vi "People Position to Steering Velocity.vi"(6 "image resolution":cluster{"x":i32, "y":i32}={"x"=640, "y"=480}, 8 "error in (no error)":errorcluster, 10 "ball pixel position":T1, 11 "ball found?":bool) -> (0 "error out":errorcluster, 3 "steering frame velocity":dbl[](array[numeric]))   [LabVIEW 2014]
doc: "This VI calculates the robot steering velocity based on the location of the tennis ball in the acquried image. If the ball is not found, then the robot will come to a stop."
uses:
  Ball Pixel Info.ctl
  Ball Tracking Globals.vi
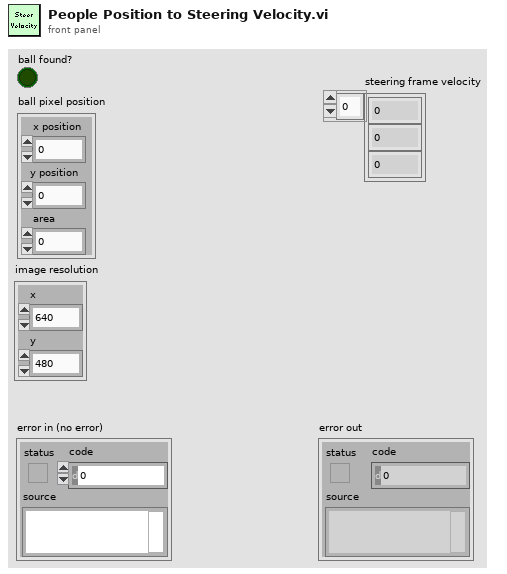
[diagram p1: front panel]
types:
  T1 = typedef "Ball Pixel Info.ctl" = cluster{"x position":dbl, "y position":dbl, "area":dbl}
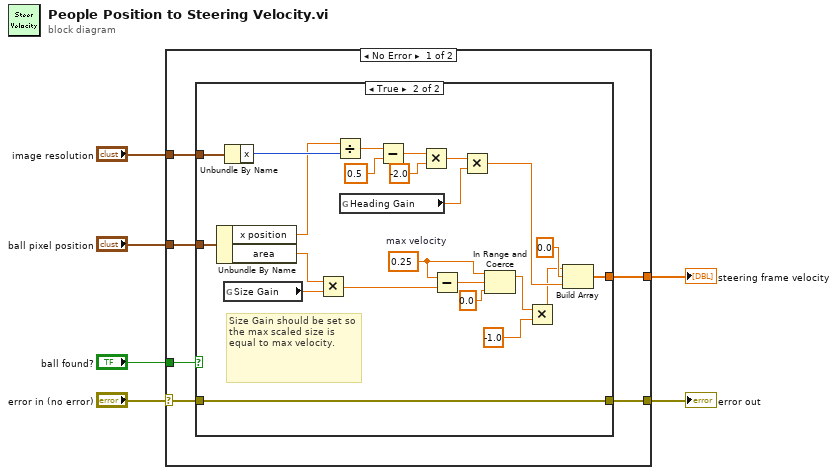
[diagram p0: block diagram]
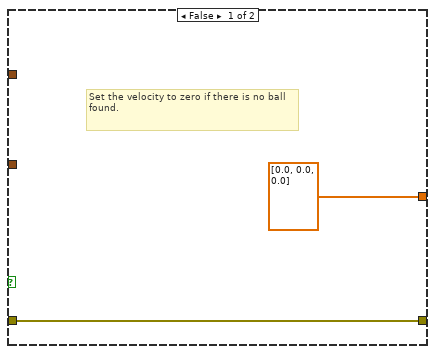
[diagram p2: hidden frame]
diagram:
  n1 = case shown="No Error" "error in (no error)" {
    selector: "error in (no error)" -> [w11 w38]
    tunnel: [w10 w38] -> w5
    tunnel: "ball found?" -> [w12 _]
    tunnel: [w9 _] -> w3
    tunnel: "ball pixel position" -> [w8 _]
    tunnel: "image resolution" -> [w7 _]
    frame No Error {
      n2 = case shown="True" w12 {
        tunnel: w11 -> [w14 w27]
        tunnel: [w14 w27] -> w10
        tunnel: [dbl[] [0.0, 0.0, 0.0] ("steering frame velocity") w31] -> w9
        tunnel: w8 -> [_ w37]
        tunnel: w7 -> [_ w30]
        frame False {
          # "Set the velocity to zero if there is no ball found."
        }
        frame True {
          w34 = 0.25  # max velocity
          # "Size Gain should be set so the max scaled size is equal to max velocity."
          n3 = Unbundle By Name(w37) -> ("x position"=w26:dbl, "area"=w36:dbl)
          n4 = global read "Ball Tracking Globals.vi" "Size Gain"() -> (w24:dbl)
          n5 = Unbundle By Name(w30) -> ("x"=w29:i32)
          n6 = Multiply(x=w36, y=w24) -> (x*y=w32:dbl)
          n7 = Divide(x=w26, y=w29) -> (x/y=w23:dbl)
          n8 = global read "Ball Tracking Globals.vi" "Heading Gain"() -> (w25:dbl)
          n9 = Subtract(x=w23, y=0.5) -> (x-y=w21:dbl)
          n10 = Multiply(x=w21, y=-2.0) -> (x*y=w19:dbl)
          n11 = Subtract(x=w34, y=w32) -> (x-y=w33:dbl)
          n12 = Multiply(x=w19, y=w25) -> (x*y=w28:dbl)
          n13 = In Range and Coerce(upper limit=w34, x=w33, lower limit=0.0) -> (coerced(x)=w17:dbl)  [unwired: 1 out]
          n14 = Multiply(x=w17, y=-1.0) -> (x*y=w15:dbl)
          n15 = Build Array(w15, 0.0, w28) -> (w31:dbl[])
        }
      }
    }
    frame Error {
    }
  }
  "error out" <- w5
  "steering frame velocity" <- w3
